vi "Heater_Enable_Chs.vi"(8 "Reload from File":bool) -> (0 "Bus Bar 4":T1={"Bus Bar"="EnFlo_Tunnel:Bus Bar 1 Enable:Y-ve Top", "Connected Items"=[]}, 1 "Bus Bar 3":T1={"Bus Bar"="EnFlo_Tunnel:Bus Bar 1 Enable:Y-ve Top", "Connected Items"=[]}, 2 "Bus Bar 2":T1={"Bus Bar"="EnFlo_Tunnel:Bus Bar 1 Enable:Y-ve Top", "Connected Items"=[]}, 3 "Bus Bar 1":T1={"Bus Bar"="EnFlo_Tunnel:Bus Bar 1 Enable:Y-ve Top", "Connected Items"=[]}, 4 "Wanted if these channels are great than zero":string[](array[string])=["EnFlo_Tunnel:Power:Chiller_Pump_Floor", "EnFlo_Tunnel:Power:Chiller_Pump_Exchanger", "EnFlo_Tunnel:Power:Exit_Heaters", "EnFlo_Tunnel:Enable:Inlet_Lamps"], 5 "Inlet Heaters":T1={"Bus Bar"="", "Connected Items"=["EnFlo_Tunnel:Enable:Inlet_Y=0_Z=50", "EnFlo_Tunnel:Enable:Inlet_Y=0_Z=150", "EnFlo_Tunnel:Enable:Inlet_Y=0_Z=250", "EnFlo_Tunnel:Enable:Inlet_Y=0_Z=350", "EnFlo_Tunnel:Enable:Inlet_Y=0_Z=450", "EnFlo_Tunnel:Enable:Inlet_Y=0_Z=550", "EnFlo_Tunnel:Enable:Inlet_Y=0_Z=650", "EnFlo_Tunnel:Enable:Inlet_Y=0_Z=750", "EnFlo_Tunnel:Enable:Inlet_Y=0_Z=850", "EnFlo_Tunnel:Enable:Inlet_Y=0_Z=950", "EnFlo_Tunnel:Enable:Inlet_Y=0_Z=1050", "EnFlo_Tunnel:Enable:Inlet_Y=0_Z=1150", "EnFlo_Tunnel:Enable:Inlet_Y=0_Z=1250", "EnFlo_Tunnel:Enable:Inlet_Y=0_Z=1350", "EnFlo_Tunnel:Enable:Inlet_Y=0_Z=1450"]})   [LabVIEW 2017]
uses:
  Anemometry/Anemometry Sub Vis/Globals/Constants_global.vi
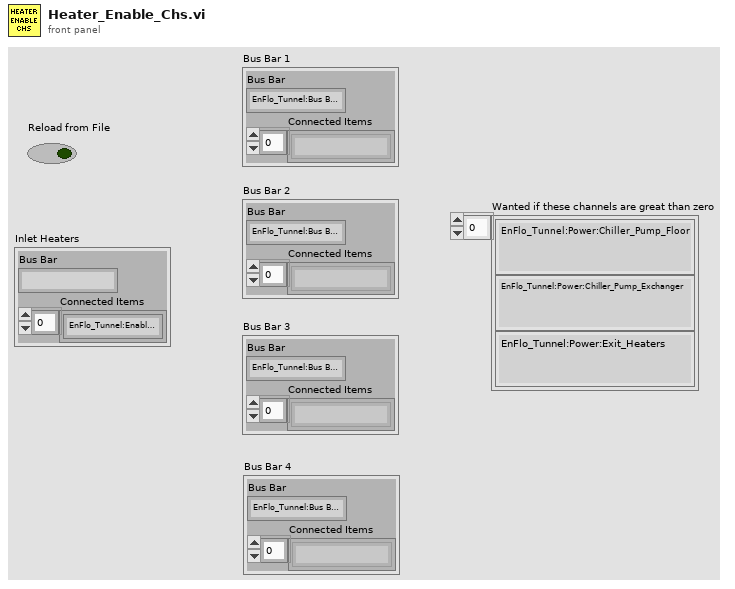
[diagram p1: front panel]
types:
  T1 = cluster{"Bus Bar":string, "Connected Items":string[]}
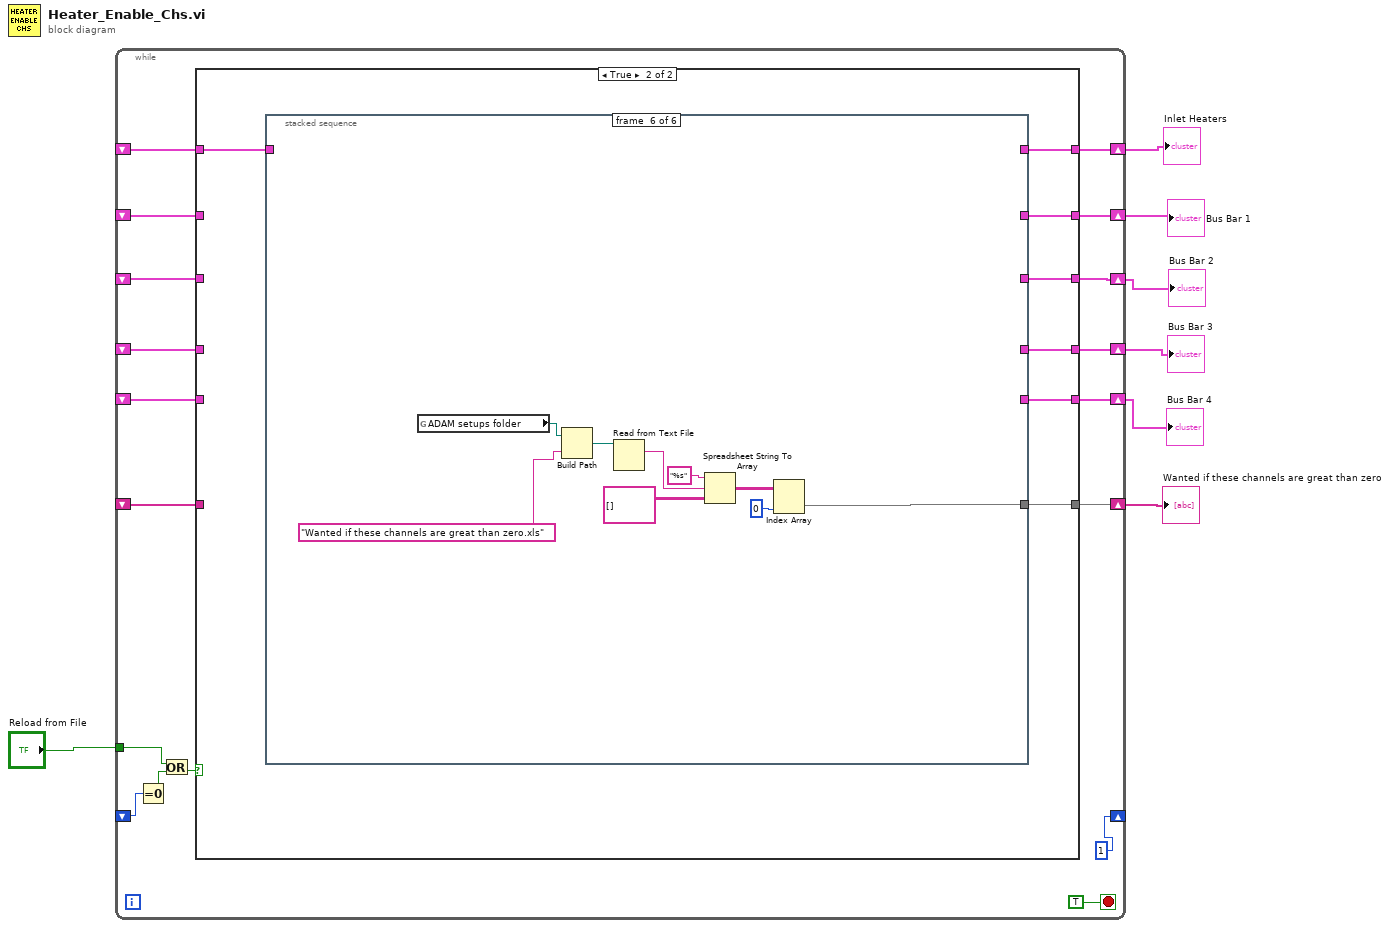
[diagram p0: block diagram]
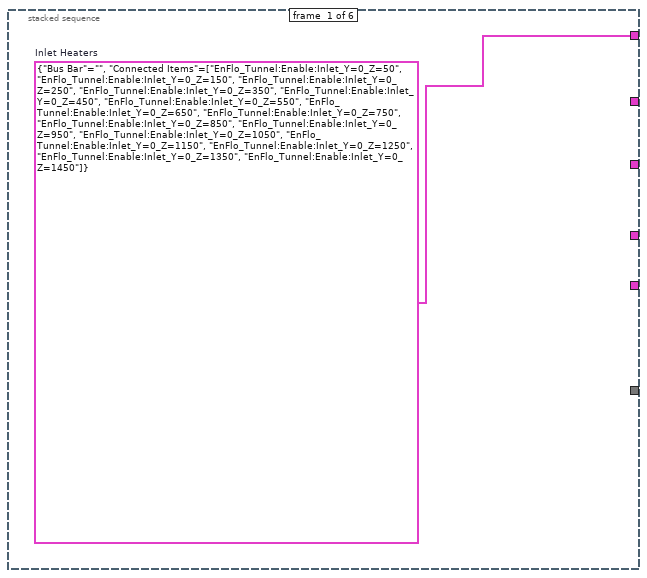
[diagram p3: hidden frame]
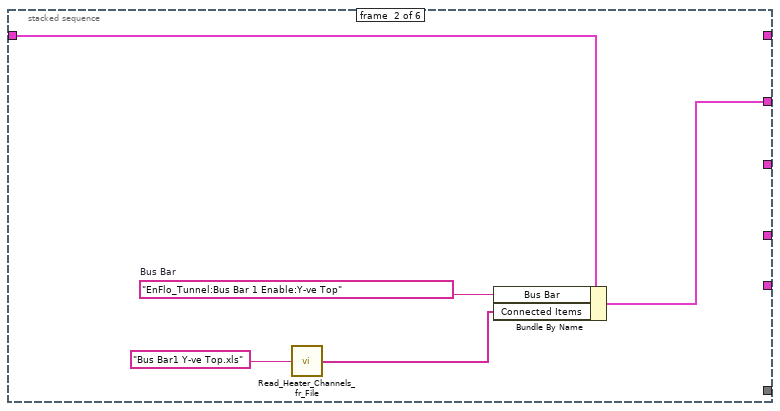
[diagram p4: hidden frame]
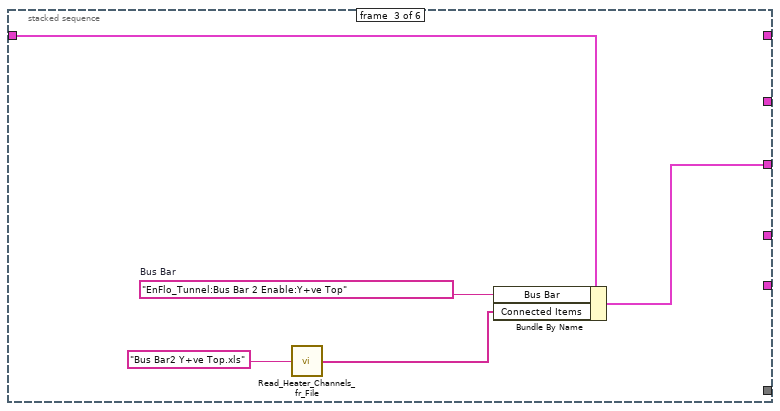
[diagram p5: hidden frame]
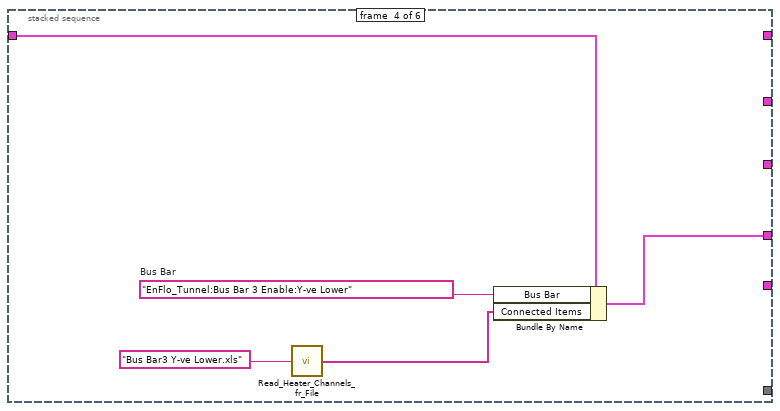
[diagram p6: hidden frame]
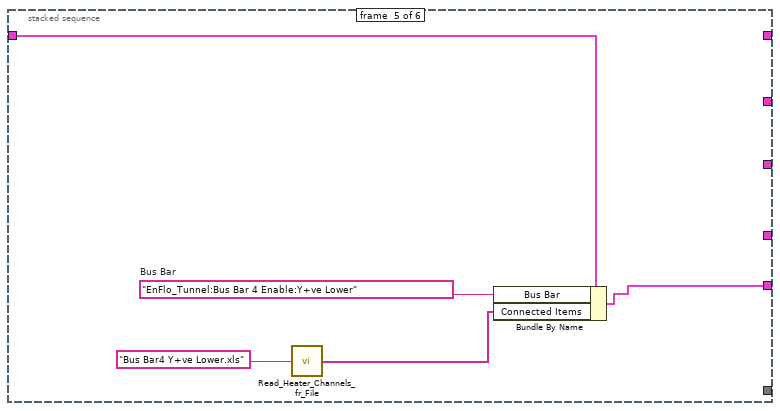
[diagram p7: hidden frame]
diagram:
  n1 = while {
    shift-right: [w22] -> w7
    shift-left: _ -> [w21]
    shift-right: [w20] -> w6
    shift-left: _ -> [w19]
    shift-right: [w18] -> w2
    shift-left: _ -> [w15]
    shift-right: [w17] -> w3
    shift-left: _ -> [w14]
    shift-right: [i16 1 ("x")] -> _
    shift-left: _ -> [w25]
    shift-right: [w16] -> w4
    shift-left: _ -> [w13]
    shift-right: [w12] -> w5
    shift-left: _ -> [w11]
    tunnel: "Reload from File" -> [w9]
    stop <- TRUE stop-if-true
    n2 = Equal To 0?(x=w25) -> (x = 0?=w24:bool)
    n3 = Or(x=w9, y=w24) -> (x .or. y?=w23:bool)
    n4 = case shown="True" w23 {
      tunnel: [w31 w38] -> w22
      tunnel: w21 -> [w31 w37]
      tunnel: [w30 w36] -> w20
      tunnel: w19 -> [w30 _]
      tunnel: [w29 w35] -> w18
      tunnel: [w28 w34] -> w17
      tunnel: [w27 w33] -> w16
      tunnel: w15 -> [w29 _]
      tunnel: w14 -> [w28 _]
      tunnel: w13 -> [w27 _]
      tunnel: [w26 w32] -> w12
      tunnel: w11 -> [w26 _]
      frame False {
      }
      frame True {
        n5 = stacked-sequence {
          tunnel: [w39 _ _ _ _ _] -> w38
          tunnel: w37 -> [_ w43 w48 w53 w58 _]
          tunnel: [_ w40 _ _ _ _] -> w36
          tunnel: [_ _ w45 _ _ _] -> w35
          tunnel: [_ _ _ w50 _ _] -> w34
          tunnel: [_ _ _ _ w55 _] -> w33
          tunnel: [_ _ _ _ _ w60] -> w32
          frame #0 {
            w39 = T1 {"Bus Bar"="", "Connected Items"=["EnFlo_Tunnel:Enable:Inlet_Y=0_Z=50", "EnFlo_Tunnel:Enable:Inlet_Y=0_Z=150", "EnFlo_Tunnel:Enable:Inlet_Y=0_Z=250", "EnFlo_Tunnel:Enable:Inlet_Y=0_Z=350", "EnFlo_Tunnel:Enable:Inlet_Y=0_Z=450", "EnFlo_Tunnel:Enable:Inlet_Y=0_Z=550", "EnFlo_Tunnel:Enable:Inlet_Y=0_Z=650", "EnFlo_Tunnel:Enable:Inlet_Y=0_Z=750", "EnFlo_Tunnel:Enable:Inlet_Y=0_Z=850", "EnFlo_Tunnel:Enable:Inlet_Y=0_Z=950", "EnFlo_Tunnel:Enable:Inlet_Y=0_Z=1050", "EnFlo_Tunnel:Enable:Inlet_Y=0_Z=1150", "EnFlo_Tunnel:Enable:Inlet_Y=0_Z=1250", "EnFlo_Tunnel:Enable:Inlet_Y=0_Z=1350", "EnFlo_Tunnel:Enable:Inlet_Y=0_Z=1450"]}  # Inlet Heaters
          }
          frame #1 {
            w42 = "EnFlo_Tunnel:Bus Bar 1 Enable:Y-ve Top"  # Bus Bar
            n6 = call "Read_Heater_Channels_fr_File.vi"("Filename"="Bus Bar1 Y-ve Top.xls" ("name or relative path")) -> ("Channel Names"=w41:string[])
            n7 = Bundle By Name(cluster=w43, "Bus Bar"=w42, "Connected Items"=w41) -> (w40:T1)
          }
          frame #2 {
            w47 = "EnFlo_Tunnel:Bus Bar 2 Enable:Y+ve Top"  # Bus Bar
            n8 = call "Read_Heater_Channels_fr_File.vi"("Filename"="Bus Bar2 Y+ve Top.xls" ("name or relative path")) -> ("Channel Names"=w46:string[])
            n9 = Bundle By Name(cluster=w48, "Bus Bar"=w47, "Connected Items"=w46) -> (w45:T1)
          }
          frame #3 {
            w52 = "EnFlo_Tunnel:Bus Bar 3 Enable:Y-ve Lower"  # Bus Bar
            n10 = call "Read_Heater_Channels_fr_File.vi"("Filename"="Bus Bar3 Y-ve Lower.xls" ("name or relative path")) -> ("Channel Names"=w51:string[])
            n11 = Bundle By Name(cluster=w53, "Bus Bar"=w52, "Connected Items"=w51) -> (w50:T1)
          }
          frame #4 {
            w57 = "EnFlo_Tunnel:Bus Bar 4 Enable:Y+ve Lower"  # Bus Bar
            n12 = call "Read_Heater_Channels_fr_File.vi"("Filename"="Bus Bar4 Y+ve Lower.xls" ("name or relative path")) -> ("Channel Names"=w56:string[])
            n13 = Bundle By Name(cluster=w58, "Bus Bar"=w57, "Connected Items"=w56) -> (w55:T1)
          }
          frame #5 {
            n14 = global read "Constants_global.vi" "ADAM setups folder"() -> (w64:path)
            n15 = Build Path(base path=w64, name or relative path="Wanted if these channels are great than zero.xls") -> (appended path=w68:path)
            n16 = Read from Text File(file (use dialog)=w68) -> (text=w67:string)  [unwired: 3 in, 3 out]
            n17 = Spreadsheet String To Array(format string="%s", spreadsheet string=w67, array type (2D Dbl)=string[][] []) -> (array=w63:string[][])  [unwired: 1 in]
            n18 = Index Array(array=w63, index (col)=0 ("disabled index (col)")) -> (element=w60:string[])  [unwired: 1 in]
          }
        }
      }
    }
  }
  "Bus Bar 2" <- w2
  "Bus Bar 4" <- w4
  "Bus Bar 3" <- w3
  "Wanted if these channels are great than zero" <- w5
  "Inlet Heaters" <- w7
  "Bus Bar 1" <- w6
